vi "reverseVersionsArray.vi"(10 "versionsArray":u8[][](array[numeric])) -> (2 "reversedVersionsArray":u8[][](array[numeric]))   [LabVIEW 2020, in "openg_variant.lvlib" / "Reflection.lvclass"]
doc: "GCraftsman JSON Object Serialization Toolkit\nwww.GCraftsman.com\nCopyright (c) 2017, GCraftsman"
uses:
  Reflection.lvclass
  Reflection.lvclass/Reflection.ctl
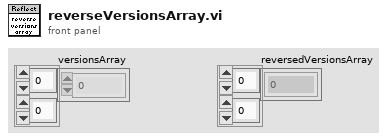
[diagram p1: front panel]
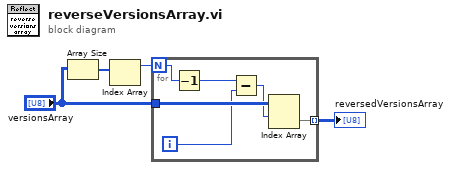
[diagram p0: block diagram]
diagram:
  n1 = Array Size(array="versionsArray") -> (size(s)=w3:i32[])
  n2 = Index Array(array=w3) -> (element=w2:i32)  [unwired: 1 in]
  n3 = for {
    N: w2 -> [w9]
    tunnel: "versionsArray" -> [w10]
    tunnel: [w5] -> w1 mode=indexing
    i -> [w7]
    n4 = Decrement(x=w9) -> (x-1=w8:i32)
    n5 = Subtract(x=w8, y=w7) -> (x-y=w6:i32)
    n6 = Index Array(array=w10, index (row)=w6) -> (element=w5:u8[])  [unwired: 1 in]
  }
  "reversedVersionsArray" <- w1
